vi "Stop Module.vi"(8 "error in (no error)":errorcluster, 9 "Wait for Module to stop? (F)":bool, 10 "Origin":string, 11 "Module ID":i32=-1) -> (0 "error out":errorcluster)   [LabVIEW 2020, in "DQMH module.lvlib"]
doc: "Send the Stop request to the Module's Main.vi.\n_____\nBased on Delacor QMH Project Template 5.0.0.82."
uses:
  DQMH module.lvlib
  Stop Argument--cluster.ctl
  <vilib>/event_ctls.llb/usereventprio.ctl
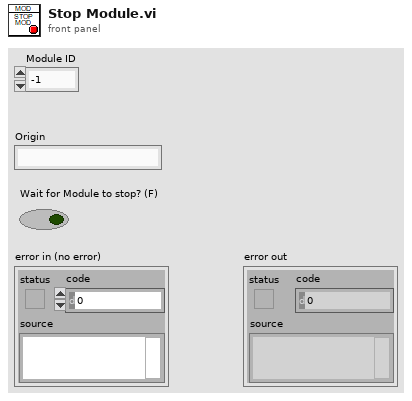
[diagram p1: front panel]
types:
  T1 = typedef "DQMH module.lvlib/Stop Argument--cluster.ctl" = cluster{"Module ID":i32, "Origin":string, "Exit via Stop Module Req?":bool, "Wait for Module to stop?":bool}
  T2 = typedef "DQMH module.lvlib/Request Events--cluster.ctl" = cluster{"Stop Module":refnum<user-event>, "Show Panel":refnum<user-event>, "Hide Panel":refnum<user-event>, "Show Diagram":refnum<user-event>, "Get Module Execution Status":refnum<user-event>, "Read ADC":refnum<user-event>, "Set Port Status":refnum<user-event>}
  T3 = typedef "usereventprio.ctl" = enum32{"high priority", "normal priority"}
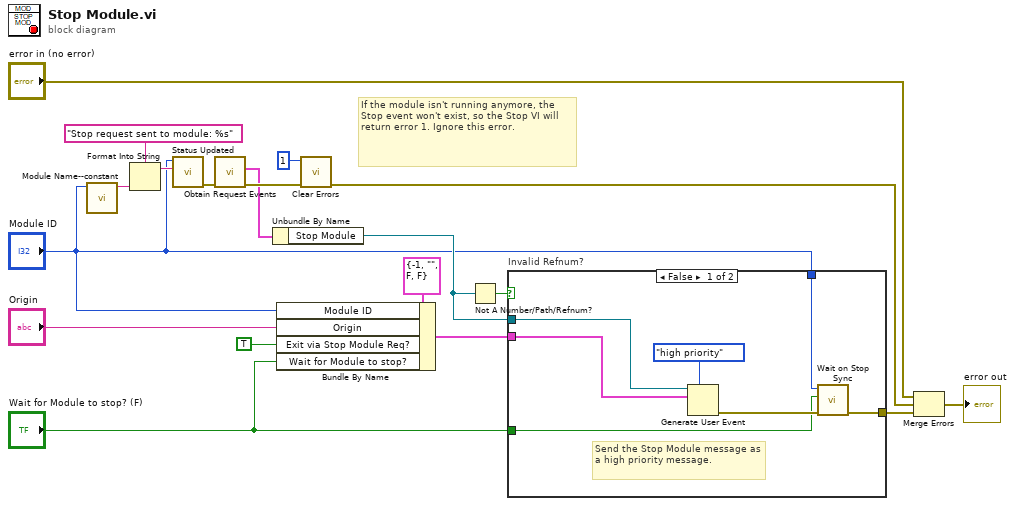
[diagram p0: block diagram]
diagram:
  # "If the module isn't running anymore, the Stop event won't exist, so the Stop VI will return error 1. Ignore this error."
  n1 = call "Module Name--constant.vi"("Module ID"="Module ID") -> ("Module Name"=w16:string)  [unwired: 10 in]
  n2 = Format Into String(format string="Stop request sent to module: %s", w16) -> (resulting string=w17:string)  [unwired: 2 in, 1 out]
  n3 = call "Status Updated.vi"("Status"=w17, "Module ID"="Module ID") -> ("error out"=w9:errorcluster)  [unwired: 9 in]
  n4 = call "Obtain Request Events.vi"("error in (no error)"=w9) -> ("error out"=w8:errorcluster, "DQMH module Request Events"=w6:T2)  [unwired: 9 in]
  n5 = Unbundle By Name(w6) -> ("Stop Module"=w11:refnum<user-event>)
  n6 = Bundle By Name(cluster=T1 {"Module ID"=-1, "Origin"="", "Exit via Stop Module Req?"=FALSE, "Wait for Module to stop?"=FALSE} ("event data"), "Module ID"="Module ID", "Origin"="Origin", "Exit via Stop Module Req?"=TRUE, "Wait for Module to stop?"="Wait for Module to stop? (F)") -> (w10:T1)
  n7 = call <vilib>:"Clear Errors.vi"("error in (no error)"=w8, "specific error code to clear (0: all)"=1) -> ("error out"=w5:errorcluster)  [unwired: 4 in, 1 out]
  n8 = Not A Number/Path/Refnum?(number/path/refnum=w11) -> (NaN/Path/Refnum?=w12:bool)
  n9 = case "Invalid Refnum?" shown="False" w12 {
    tunnel: [w22 _] -> w4
    tunnel: w10 -> [w26 _]
    tunnel: w11 -> [w25 _]
    tunnel: "Module ID" -> [w21 _]
    tunnel: "Wait for Module to stop? (F)" -> [w20 _]
    frame False {
      # "Send the Stop Module message as a high priority message."
      n10 = Generate User Event(priority (normal)=usereventprio."high priority", user event=w25, event data cluster=w26) -> (error out=w23:errorcluster)  [unwired: 1 in, 1 out]
      n11 = call "Wait on Stop Sync.vi"("error in (no error)"=w23, "Wait for Module to stop?"=w20, "Module ID"=w21) -> ("error out"=w22:errorcluster)  [unwired: 8 in]
    }
    frame True {
      # "Module is exiting. No need to send the standard \"not running\" error that is sent in other request VIs."
    }
  }
  n12 = Merge Errors("error in (no error)", w5, w4) -> (→"error out":errorcluster)
